vi "首页.vi"() -> ()   [LabVIEW 2016]
uses:
  <vilib>/Utility/miscctls.llb/LVPointTypeDef.ctl
  <vilib>/addons/database/_DB Variant To Data/Database Variant To Data.xnode
  PLC/PLC.lvlib
panel:
  out "大项目框 12":T1(xcontrol)
  out "大项目框 11":T1(xcontrol)
  out "大项目框 10":T1(xcontrol)
  out "大项目框 9":T1(xcontrol)
  out "大项目框 8":T1(xcontrol)
  out "大项目框 7":T1(xcontrol)
  out "大项目框 6":T1(xcontrol)
  out "大项目框 5":T1(xcontrol)
  out "大项目框 4":T1(xcontrol)
  out "大项目框 3":T1(xcontrol)
  out "大项目框 2":T1(xcontrol)
  out "大项目框":T1(xcontrol)
  out "湿度":string="75.5 %"
  out "室温":string="25.8 ℃"
  # "室温:"
  # "湿度:"
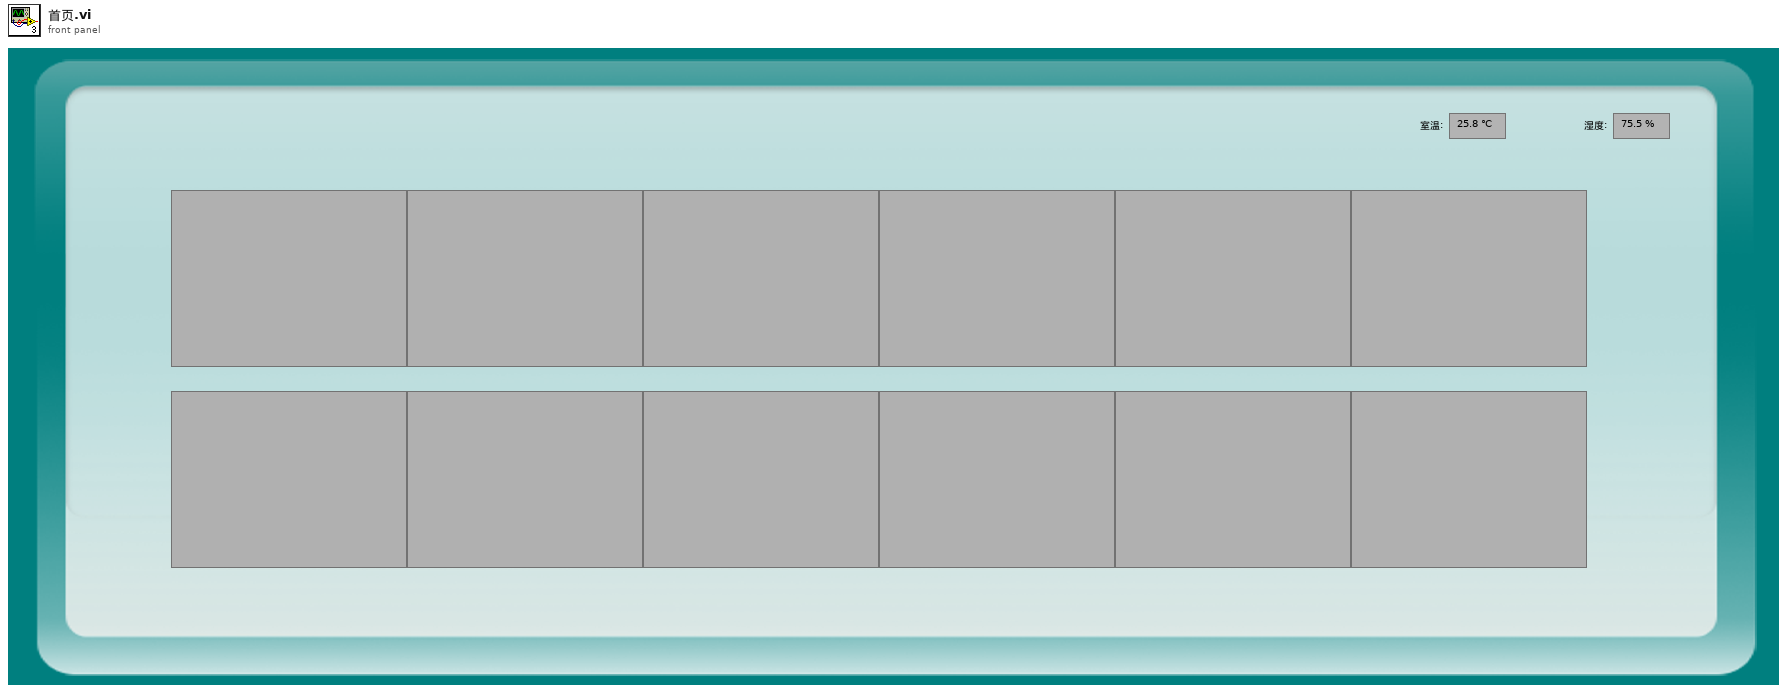
[diagram p1: front panel]
types:
  T1 = cluster{"中文项目名称":string, "英文项目名称":string, "单位":string, "浓度值":string}
  T2 = typedef "LVPointTypeDef.ctl" = cluster{"Horizontal":i16, "Vertical":i16}
  T3 = cluster{"显示参数中文名":string, "显示参数英文名":string, "显示浓度":string, "显示单位":string}[]
  T4 = cluster{"显示参数中文名":string, "显示参数英文名":string, "显示浓度":string, "显示单位":string}
  T5 = cluster{"水温":bool, "pH":bool, "DO":bool, "Cond":bool, "Turb":bool, "氨氮":bool, "总磷":bool, "总氮":bool, "CODMn":bool, "CODCr":bool, "水位":bool, "流速":bool, "瞬时流量":bool, "室温":bool, "湿度":bool}
  T6 = cluster{"AD0":sgl, "AD1":sgl, "AD2":sgl, "AD3":sgl, "AD4":sgl, "AD5":sgl}
  T7 = typedef "LVDateTimeRec.ctl" = cluster{"秒数的小数部分":dbl, "秒":i32, "分":i32, "时":i32, "日":i32, "月":i32, "年":i32, "天数（周）":i32, "天数（年）":i32, "DST":i32}
  T8 = cluster{"时间标识":timestamp, "监测值":sgl, "单位":string}
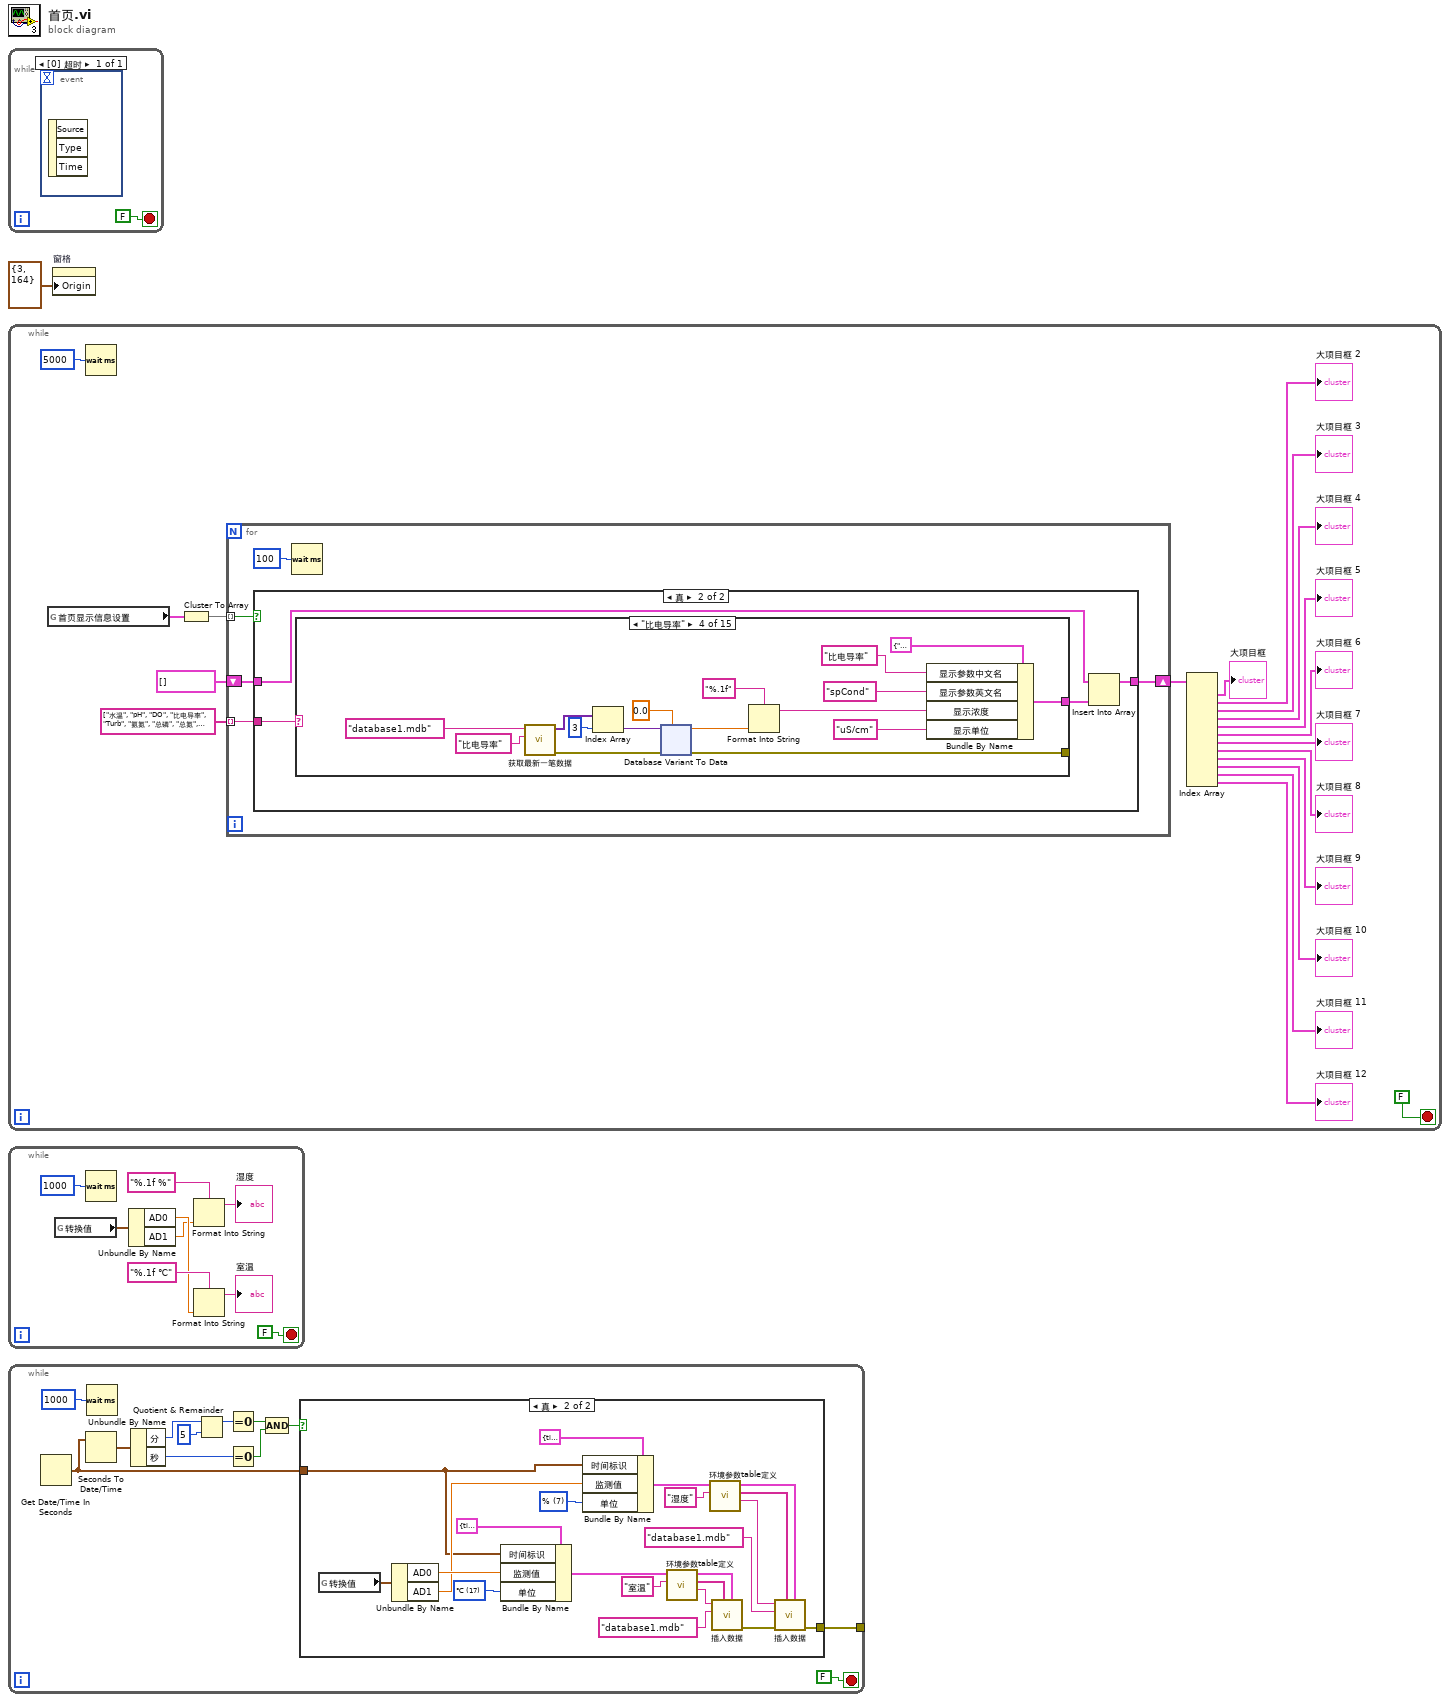
[diagram p0: block diagram]
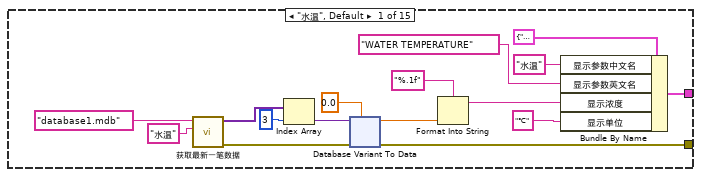
[diagram p4: hidden frame]
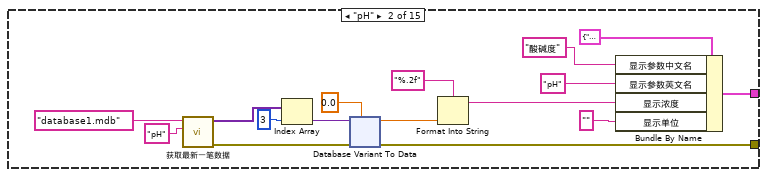
[diagram p5: hidden frame]
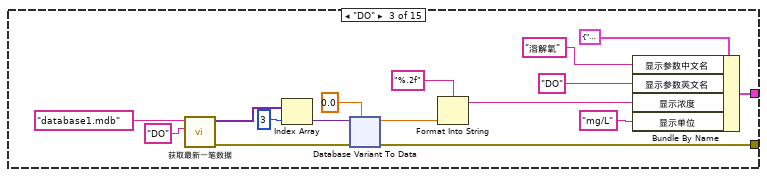
[diagram p6: hidden frame]
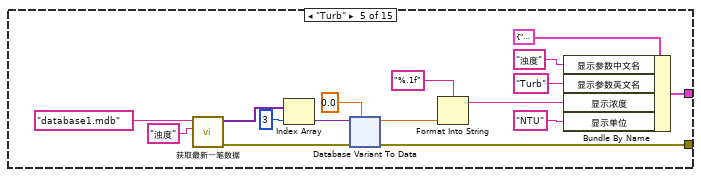
[diagram p7: hidden frame]
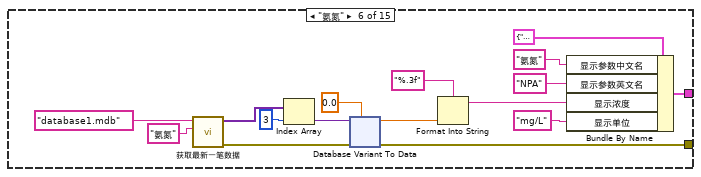
[diagram p8: hidden frame]
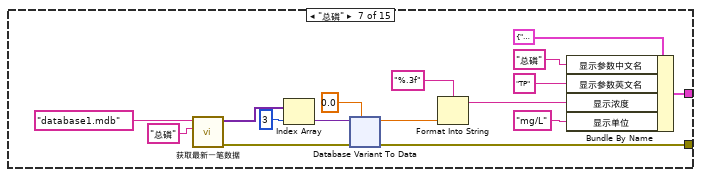
[diagram p9: hidden frame]
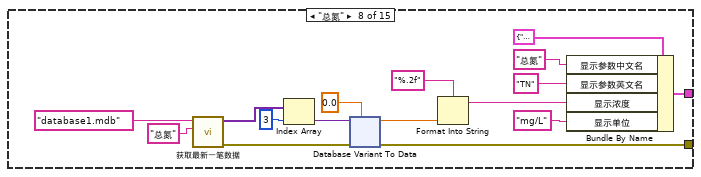
[diagram p10: hidden frame]
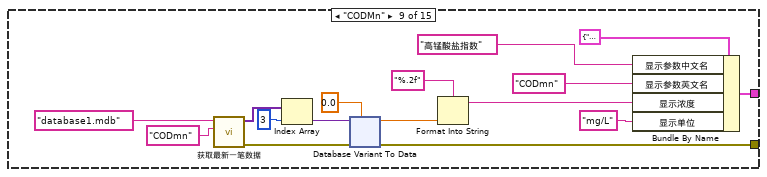
[diagram p11: hidden frame]
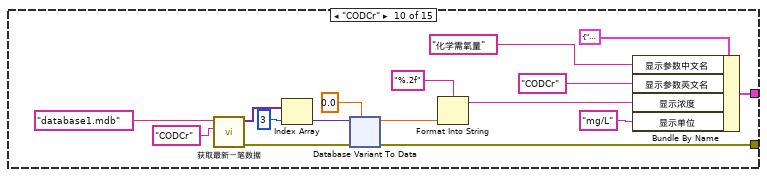
[diagram p12: hidden frame]
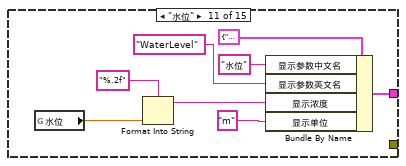
[diagram p13: hidden frame]
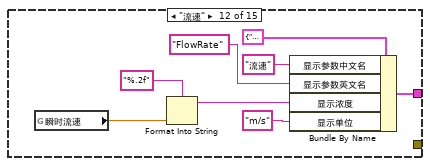
[diagram p14: hidden frame]
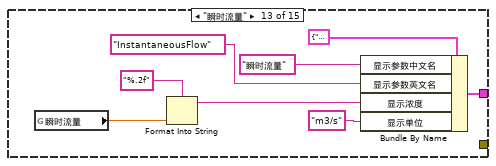
[diagram p15: hidden frame]
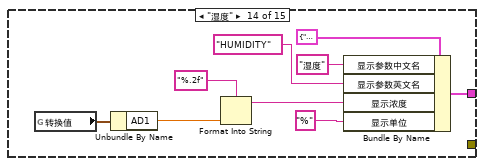
[diagram p16: hidden frame]
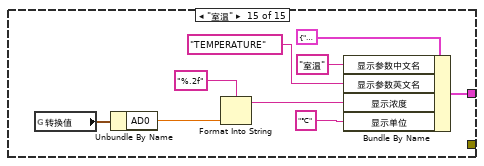
[diagram p17: hidden frame]
diagram:
  n1 = while {
    stop <- FALSE stop-if-true
    n2 = event shown="[0] 超时" {
      selector: _ -> [_]
      dyn-events: _ -> [_]
      timeout: _ -> [_]
      event Timeout {
        n3 = event-data() -> ()  [unwired: 1 in, 3 out]
      }
    }
  }
  n4 = while {
    stop <- FALSE stop-if-true
    n5 = global read "系统设置全局变量.vi" "首页显示信息设置"() -> (w4:T5)
    n6 = Wait (ms)(milliseconds to wait=u32 5000 ("等待时间（毫秒）")) -> ()  [unwired: 1 out]
    n7 = Cluster To Array(cluster=w4) -> (array=w3:bool[])
    n8 = for {
      tunnel: w3 -> [w26] mode=indexing
      tunnel: string[] ["水温", "pH", "DO", "比电导率", "Turb", "氨氮", "总磷", "总氮", "CODMn", "CODCr", "水位", "流速", "瞬时流量"] -> [w25] mode=indexing
      shift-right: [w23] -> w18
      shift-left: T3 [] -> [w24]
      n9 = case shown="真" w26 {
        tunnel: w25 -> [_ w31]
        tunnel: w24 -> [w27 w30]
        tunnel: [w27 w29] -> w23
        frame False {
        }
        frame True {
          n10 = case shown="\"比电导率\"" w31 {
            tunnel: [w32 w91 w139 w187 w235 w283 w331 w379 w427 w475 w515 w523 w528 w540 w549] -> w28
            tunnel: [w33 w80 w128 w176 w224 w272 w320 w368 w416 w464 _ _ _ _ _] -> _
            frame "水温", Default {
              n11 = call "获取最新一笔数据.vi"("table"="水温", "database"="database1.mdb" ("名称或相对路径")) -> ("error out"=w34:errorcluster, "子数组"=w40:variant[])  [unwired: 8 in]
              n12 = Index Array(array=w40, index=3 ("索引")) -> (element=w38:variant)
              n13 = xnode "Database Variant To Data"("database variant"=w38, "error in (no error)"=w34, "type"=0.0) -> ("data"=w35:dbl, "error out"=w33:errorcluster)
              n14 = Format Into String(format string="%.1f" ("格式字符串"), w35) -> (resulting string=w42:string)  [unwired: 2 in, 1 out]
              n15 = Bundle By Name(cluster=T4 {"显示参数中文名"="", "显示参数英文名"="", "显示浓度"="", "显示单位"=""} ("元素"), "显示参数中文名"="水温", "显示参数英文名"="WATER TEMPERATURE", "显示浓度"=w42, "显示单位"="℃") -> (w32:T4)
            }
            frame "pH" {
              n16 = call "获取最新一笔数据.vi"("table"="pH", "database"="database1.mdb" ("名称或相对路径")) -> ("error out"=w81:errorcluster, "子数组"=w87:variant[])  [unwired: 8 in]
              n17 = Index Array(array=w87, index=3 ("索引")) -> (element=w85:variant)
              n18 = xnode "Database Variant To Data"("database variant"=w85, "error in (no error)"=w81, "type"=0.0) -> ("data"=w82:dbl, "error out"=w80:errorcluster)
              n19 = Format Into String(format string="%.2f" ("格式字符串"), w82) -> (resulting string=w89:string)  [unwired: 2 in, 1 out]
              n20 = Bundle By Name(cluster=T4 {"显示参数中文名"="", "显示参数英文名"="", "显示浓度"="", "显示单位"=""} ("元素"), "显示参数中文名"="酸碱度", "显示参数英文名"="pH", "显示浓度"=w89, "显示单位"="") -> (w91:T4)
            }
            frame "DO" {
              n21 = call "获取最新一笔数据.vi"("table"="DO", "database"="database1.mdb" ("名称或相对路径")) -> ("error out"=w129:errorcluster, "子数组"=w135:variant[])  [unwired: 8 in]
              n22 = Index Array(array=w135, index=3 ("索引")) -> (element=w133:variant)
              n23 = xnode "Database Variant To Data"("database variant"=w133, "error in (no error)"=w129, "type"=0.0) -> ("data"=w130:dbl, "error out"=w128:errorcluster)
              n24 = Format Into String(format string="%.2f" ("格式字符串"), w130) -> (resulting string=w137:string)  [unwired: 2 in, 1 out]
              n25 = Bundle By Name(cluster=T4 {"显示参数中文名"="", "显示参数英文名"="", "显示浓度"="", "显示单位"=""} ("元素"), "显示参数中文名"="溶解氧", "显示参数英文名"="DO", "显示浓度"=w137, "显示单位"="mg/L") -> (w139:T4)
            }
            frame "比电导率" {
              n26 = call "获取最新一笔数据.vi"("table"="比电导率", "database"="database1.mdb" ("名称或相对路径")) -> ("error out"=w177:errorcluster, "子数组"=w183:variant[])  [unwired: 8 in]
              n27 = Index Array(array=w183, index=3 ("索引")) -> (element=w181:variant)
              n28 = xnode "Database Variant To Data"("database variant"=w181, "error in (no error)"=w177, "type"=0.0) -> ("data"=w178:dbl, "error out"=w176:errorcluster)
              n29 = Format Into String(format string="%.1f" ("格式字符串"), w178) -> (resulting string=w185:string)  [unwired: 2 in, 1 out]
              n30 = Bundle By Name(cluster=T4 {"显示参数中文名"="", "显示参数英文名"="", "显示浓度"="", "显示单位"=""} ("元素"), "显示参数中文名"="比电导率", "显示参数英文名"="spCond", "显示浓度"=w185, "显示单位"="uS/cm") -> (w187:T4)
            }
            frame "Turb" {
              n31 = call "获取最新一笔数据.vi"("table"="浊度", "database"="database1.mdb" ("名称或相对路径")) -> ("error out"=w225:errorcluster, "子数组"=w231:variant[])  [unwired: 8 in]
              n32 = Index Array(array=w231, index=3 ("索引")) -> (element=w229:variant)
              n33 = xnode "Database Variant To Data"("database variant"=w229, "error in (no error)"=w225, "type"=0.0) -> ("data"=w226:dbl, "error out"=w224:errorcluster)
              n34 = Format Into String(format string="%.1f" ("格式字符串"), w226) -> (resulting string=w233:string)  [unwired: 2 in, 1 out]
              n35 = Bundle By Name(cluster=T4 {"显示参数中文名"="", "显示参数英文名"="", "显示浓度"="", "显示单位"=""} ("元素"), "显示参数中文名"="浊度", "显示参数英文名"="Turb", "显示浓度"=w233, "显示单位"="NTU") -> (w235:T4)
            }
            frame "氨氮" {
              n36 = call "获取最新一笔数据.vi"("table"="氨氮", "database"="database1.mdb" ("名称或相对路径")) -> ("error out"=w273:errorcluster, "子数组"=w279:variant[])  [unwired: 8 in]
              n37 = Index Array(array=w279, index=3 ("索引")) -> (element=w277:variant)
              n38 = xnode "Database Variant To Data"("database variant"=w277, "error in (no error)"=w273, "type"=0.0) -> ("data"=w274:dbl, "error out"=w272:errorcluster)
              n39 = Format Into String(format string="%.3f" ("格式字符串"), w274) -> (resulting string=w281:string)  [unwired: 2 in, 1 out]
              n40 = Bundle By Name(cluster=T4 {"显示参数中文名"="", "显示参数英文名"="", "显示浓度"="", "显示单位"=""} ("元素"), "显示参数中文名"="氨氮", "显示参数英文名"="NPA", "显示浓度"=w281, "显示单位"="mg/L") -> (w283:T4)
            }
            frame "总磷" {
              n41 = call "获取最新一笔数据.vi"("table"="总磷", "database"="database1.mdb" ("名称或相对路径")) -> ("error out"=w321:errorcluster, "子数组"=w327:variant[])  [unwired: 8 in]
              n42 = Index Array(array=w327, index=3 ("索引")) -> (element=w325:variant)
              n43 = xnode "Database Variant To Data"("database variant"=w325, "error in (no error)"=w321, "type"=0.0) -> ("data"=w322:dbl, "error out"=w320:errorcluster)
              n44 = Format Into String(format string="%.3f" ("格式字符串"), w322) -> (resulting string=w329:string)  [unwired: 2 in, 1 out]
              n45 = Bundle By Name(cluster=T4 {"显示参数中文名"="", "显示参数英文名"="", "显示浓度"="", "显示单位"=""} ("元素"), "显示参数中文名"="总磷", "显示参数英文名"="TP", "显示浓度"=w329, "显示单位"="mg/L") -> (w331:T4)
            }
            frame "总氮" {
              n46 = call "获取最新一笔数据.vi"("table"="总氮", "database"="database1.mdb" ("名称或相对路径")) -> ("error out"=w369:errorcluster, "子数组"=w375:variant[])  [unwired: 8 in]
              n47 = Index Array(array=w375, index=3 ("索引")) -> (element=w373:variant)
              n48 = xnode "Database Variant To Data"("database variant"=w373, "error in (no error)"=w369, "type"=0.0) -> ("data"=w370:dbl, "error out"=w368:errorcluster)
              n49 = Format Into String(format string="%.2f" ("格式字符串"), w370) -> (resulting string=w377:string)  [unwired: 2 in, 1 out]
              n50 = Bundle By Name(cluster=T4 {"显示参数中文名"="", "显示参数英文名"="", "显示浓度"="", "显示单位"=""} ("元素"), "显示参数中文名"="总氮", "显示参数英文名"="TN", "显示浓度"=w377, "显示单位"="mg/L") -> (w379:T4)
            }
            frame "CODMn" {
              n51 = call "获取最新一笔数据.vi"("table"="CODmn", "database"="database1.mdb" ("名称或相对路径")) -> ("error out"=w417:errorcluster, "子数组"=w423:variant[])  [unwired: 8 in]
              n52 = Index Array(array=w423, index=3 ("索引")) -> (element=w421:variant)
              n53 = xnode "Database Variant To Data"("database variant"=w421, "error in (no error)"=w417, "type"=0.0) -> ("data"=w418:dbl, "error out"=w416:errorcluster)
              n54 = Format Into String(format string="%.2f" ("格式字符串"), w418) -> (resulting string=w425:string)  [unwired: 2 in, 1 out]
              n55 = Bundle By Name(cluster=T4 {"显示参数中文名"="", "显示参数英文名"="", "显示浓度"="", "显示单位"=""} ("元素"), "显示参数中文名"="高锰酸盐指数", "显示参数英文名"="CODmn", "显示浓度"=w425, "显示单位"="mg/L") -> (w427:T4)
            }
            frame "CODCr" {
              n56 = call "获取最新一笔数据.vi"("table"="CODCr", "database"="database1.mdb" ("名称或相对路径")) -> ("error out"=w465:errorcluster, "子数组"=w471:variant[])  [unwired: 8 in]
              n57 = Index Array(array=w471, index=3 ("索引")) -> (element=w469:variant)
              n58 = xnode "Database Variant To Data"("database variant"=w469, "error in (no error)"=w465, "type"=0.0) -> ("data"=w466:dbl, "error out"=w464:errorcluster)
              n59 = Format Into String(format string="%.2f" ("格式字符串"), w466) -> (resulting string=w473:string)  [unwired: 2 in, 1 out]
              n60 = Bundle By Name(cluster=T4 {"显示参数中文名"="", "显示参数英文名"="", "显示浓度"="", "显示单位"=""} ("元素"), "显示参数中文名"="化学需氧量", "显示参数英文名"="CODCr", "显示浓度"=w473, "显示单位"="mg/L") -> (w475:T4)
            }
            frame "水位" {
              n61 = global read "流量计全局变量.vi" "水位"() -> (w512:dbl)
              n62 = Format Into String(format string="%.2f" ("格式字符串"), w512) -> (resulting string=w513:string)  [unwired: 2 in, 1 out]
              n63 = Bundle By Name(cluster=T4 {"显示参数中文名"="", "显示参数英文名"="", "显示浓度"="", "显示单位"=""} ("元素"), "显示参数中文名"="水位", "显示参数英文名"="WaterLevel", "显示浓度"=w513, "显示单位"="m") -> (w515:T4)
            }
            frame "流速" {
              n64 = global read "流量计全局变量.vi" "瞬时流速"() -> (w520:dbl)
              n65 = Format Into String(format string="%.2f" ("格式字符串"), w520) -> (resulting string=w521:string)  [unwired: 2 in, 1 out]
              n66 = Bundle By Name(cluster=T4 {"显示参数中文名"="", "显示参数英文名"="", "显示浓度"="", "显示单位"=""} ("元素"), "显示参数中文名"="流速", "显示参数英文名"="FlowRate", "显示浓度"=w521, "显示单位"="m/s") -> (w523:T4)
            }
            frame "瞬时流量" {
              n67 = global read "流量计全局变量.vi" "瞬时流量"() -> (w529:dbl)
              n68 = Format Into String(format string="%.2f" ("格式字符串"), w529) -> (resulting string=w530:string)  [unwired: 2 in, 1 out]
              n69 = Bundle By Name(cluster=T4 {"显示参数中文名"="", "显示参数英文名"="", "显示浓度"="", "显示单位"=""} ("元素"), "显示参数中文名"="瞬时流量", "显示参数英文名"="InstantaneousFlow", "显示浓度"=w530, "显示单位"="m3/s") -> (w528:T4)
            }
            frame "湿度" {
              n70 = global read "采配水全局变量.vi" "转换值"() -> (w537:T6)
              n71 = Unbundle By Name(w537) -> ("AD1"=w539:sgl)
              n72 = Format Into String(format string="%.2f" ("格式字符串"), w539) -> (resulting string=w536:string)  [unwired: 2 in, 1 out]
              n73 = Bundle By Name(cluster=T4 {"显示参数中文名"="", "显示参数英文名"="", "显示浓度"="", "显示单位"=""} ("元素"), "显示参数中文名"="湿度", "显示参数英文名"="HUMIDITY", "显示浓度"=w536, "显示单位"="%") -> (w540:T4)
            }
            frame "室温" {
              n74 = global read "采配水全局变量.vi" "转换值"() -> (w546:T6)
              n75 = Unbundle By Name(w546) -> ("AD0"=w548:sgl)
              n76 = Format Into String(format string="%.2f" ("格式字符串"), w548) -> (resulting string=w545:string)  [unwired: 2 in, 1 out]
              n77 = Bundle By Name(cluster=T4 {"显示参数中文名"="", "显示参数英文名"="", "显示浓度"="", "显示单位"=""} ("元素"), "显示参数中文名"="室温", "显示参数英文名"="TEMPERATURE", "显示浓度"=w545, "显示单位"="℃") -> (w549:T4)
            }
          }
          n78 = Insert Into Array(array=w30, new element=w28) -> (w29:T3)  [unwired: 1 in]
        }
      }
      n79 = Wait (ms)(milliseconds to wait=u32 100 ("等待时间（毫秒）")) -> ()  [unwired: 1 out]
    }
    n80 = Index Array(array=w18) -> (element #1=→"大项目框":T4, element #2=→"大项目框 2":T4, element #3=→"大项目框 3":T4, element #4=→"大项目框 4":T4, element #5=→"大项目框 5":T4, element #6=→"大项目框 6":T4, element #7=→"大项目框 7":T4, element #8=→"大项目框 8":T4, element #9=→"大项目框 9":T4, element #10=→"大项目框 10":T4, element #11=→"大项目框 11":T4, element #12=→"大项目框 12":T4)  [unwired: 12 in]
  }
  n81 = while {
    stop <- FALSE stop-if-true
    n82 = global read "采配水全局变量.vi" "转换值"() -> (w560:T6)
    n83 = Wait (ms)(milliseconds to wait=u32 1000 ("等待时间（毫秒）")) -> ()  [unwired: 1 out]
    n84 = Unbundle By Name(w560) -> ("AD0"=w555:sgl, "AD1"=w554:sgl)
    n85 = Format Into String(format string="%.1f %" ("格式字符串"), w554) -> (resulting string=→"湿度":string)  [unwired: 2 in, 1 out]
    n86 = Format Into String(format string="%.1f ℃" ("格式字符串"), w555) -> (resulting string=→"室温":string)  [unwired: 2 in, 1 out]
  }
  n87 = while {
    tunnel: [w573] -> _
    stop <- FALSE stop-if-true
    n88 = Get Date/Time In Seconds() -> (seconds since 1Jan1904=w572:timestamp)
    n89 = Seconds To Date/Time(time stamp (now)=w572) -> (date time rec=w571:T7)  [unwired: 1 in]
    n90 = Wait (ms)(milliseconds to wait=u32 1000 ("等待时间（毫秒）")) -> ()  [unwired: 1 out]
    n91 = Unbundle By Name(w571) -> ("分"=w570:i32, "秒"=w568:i32)
    n92 = Quotient & Remainder(x=w570, y=5) -> (x-y*floor(x/y)=w567:i32)  [unwired: 1 out]
    n93 = Equal To 0?(x=w567) -> (x = 0?=w566:bool)
    n94 = Equal To 0?(x=w568) -> (x = 0?=w565:bool)
    n95 = Compound Arithmetic op=AND ("复合运算")(w566, w565) -> (w564:bool)
    n96 = case shown="真" w564 {
      tunnel: [_ w588] -> w573
      tunnel: w572 -> [_ w576]
      frame False {
      }
      frame True {
        w581 = u16 7 items=["ug/L", "mg/L", "ppm", "mg/m3", "cm", "ppb", "ug/m3", "%", "nmol/mol", "umol/mol", "MPN/L", "MPN/100ml", "ng/m3", "NTU", "无量纲", "ms/cm", "us/cm", "℃", "V"] ("单位")
        w585 = u16 17 items=["ug/L", "mg/L", "ppm", "mg/m3", "cm", "ppb", "ug/m3", "%", "nmol/mol", "umol/mol", "MPN/L", "MPN/100ml", "ng/m3", "NTU", "无量纲", "ms/cm", "us/cm", "℃", "V"] ("单位")
        n97 = global read "采配水全局变量.vi" "转换值"() -> (w596:T6)
        n98 = Unbundle By Name(w596) -> ("AD0"=w584:sgl, "AD1"=w582:sgl)
        n99 = Bundle By Name(cluster=cluster{"时间标识":timestamp, "监测值":sgl, "单位":u16} {"时间标识"=timestamp(0 s since 1904-01-01), "监测值"=0.0, "单位"=0} ("data"), "时间标识"=w576, "监测值"=w584, "单位"=w585) -> (w586:cluster{"时间标识":timestamp, "监测值":sgl, "单位":u16})
        n100 = Bundle By Name(cluster=cluster{"时间标识":timestamp, "监测值":sgl, "单位":u16} {"时间标识"=timestamp(0 s since 1904-01-01), "监测值"=0.0, "单位"=0} ("data"), "时间标识"=w576, "监测值"=w582, "单位"=w581) -> (w580:cluster{"时间标识":timestamp, "监测值":sgl, "单位":u16})
        n101 = call "环境参数table定义.vi"("table 输入"="室温", "data"=w586) -> ("table 输出"=w595:string, "columns"=w594:string[], "data输出"=w593:T8)  [unwired: 7 in]
        n102 = call "环境参数table定义.vi"("table 输入"="湿度", "data"=w580) -> ("table 输出"=w590:string, "columns"=w591:string[], "data输出"=w592:T8)  [unwired: 7 in]
        n103 = call "插入数据.vi"("data"=w593, "columns"=w594, "database"="database1.mdb" ("table 输入"), "table"=w595) -> ("error out"=w589:errorcluster)  [unwired: 7 in]
        n104 = call "插入数据.vi"("data"=w592, "columns"=w591, "error in (no error)"=w589, "database"="database1.mdb" ("table 输入"), "table"=w590) -> ("error out"=w588:errorcluster)  [unwired: 6 in]
      }
    }
  }
  n105 = property on="窗格" class="Pane"("Origin"=T2 {"Horizontal"=3, "Vertical"=164} ("原点")) -> ()  [unwired: 2 in, 2 out]
